vi "Remove UI without races.vi"(8 "error in":errorcluster, 10 "standard events":T1, 11 "sub panel ref in":refnum<vi>) -> (0 "error out":errorcluster, 3 "sub panel ref out":refnum<vi>)   [LabVIEW 2013, in "configuration library.lvlib"]
uses:
  configuration library.lvlib
  <vilib>/NI/Configuration Framework/Node/StandardEvents.ctl
  <vilib>/NI/Configuration Framework/Node/UserEventRef.ctl
  <vilib>/NI/Configuration Framework/Controls/EventCluster.ctl
  <vilib>/NI/Configuration Framework/Node/NodeChangeEvent.ctl
  <vilib>/NI/Configuration Framework/Node/NodeRef.ctl
  <vilib>/NI/Configuration Framework/Node/NISE_CEF_Node.lvclass
  <vilib>/NI/Configuration Framework/Node/CacheState.ctl
  <vilib>/NI/Configuration Framework/Node/RefreshUIEvent.ctl
  <vilib>/NI/Configuration Framework/Node/StopEvent.ctl
  <vilib>/NI/Configuration Framework/NISE_CEF_TreeControl.lvlib
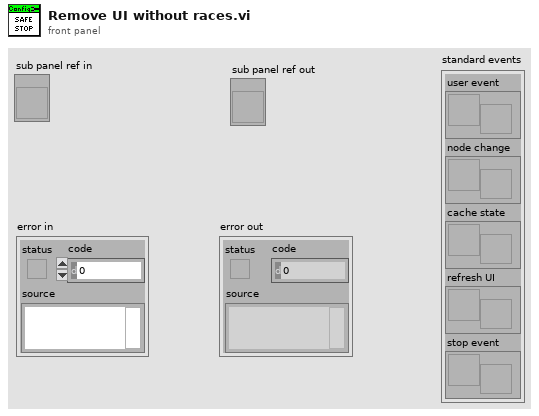
[diagram p1: front panel]
types:
  T1 = typedef "NISE_CEF_Node.lvclass/StandardEvents.ctl" = cluster{"user event":T2, "node change":T3, "cache state":T4, "refresh UI":T5, "stop event":T6}
  T2 = typedef "NISE_CEF_Node.lvclass/UserEventRef.ctl" = refnum<user-event>
  T3 = typedef "NISE_CEF_Node.lvclass/NodeChangeEvent.ctl" = refnum<user-event>
  T4 = typedef "NISE_CEF_Node.lvclass/CacheState.ctl" = refnum<user-event>
  T5 = typedef "NISE_CEF_Node.lvclass/RefreshUIEvent.ctl" = refnum<user-event>
  T6 = typedef "NISE_CEF_Node.lvclass/StopEvent.ctl" = refnum<user-event>
  T7 = typedef "NISE_CEF_TreeControl.lvlib/EventCluster.ctl" = cluster{"command":string, "data":string}
  T8 = enum32{"Bad", "Idle", "Run top level", "Running"}
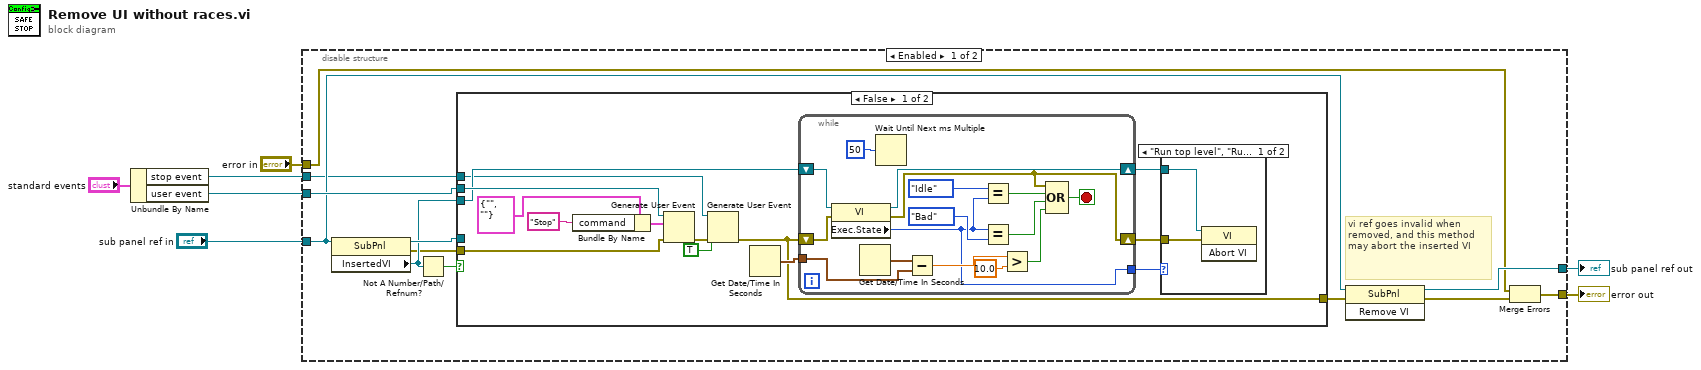
[diagram p0: block diagram]
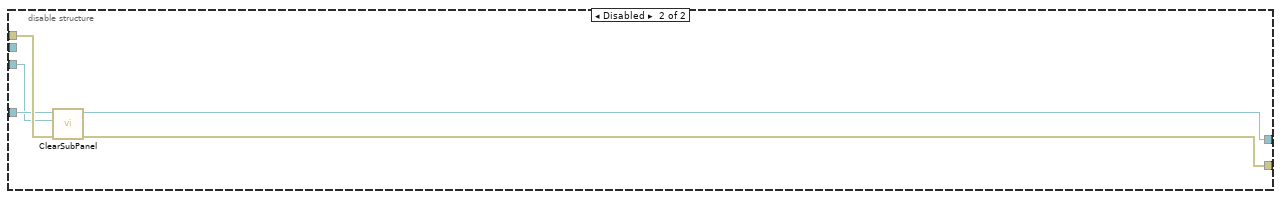
[diagram p4: hidden frame]
diagram:
  n1 = Unbundle By Name("standard events") -> ("stop event"=w1:T6, "user event"=w2:T2)
  n2 = disable-structure shown="Enabled" {
    disable-tunnel: "error in" -> [w12 w57]
    disable-tunnel: "sub panel ref in" -> [w14 w56]
    disable-tunnel: w2 -> [w18 w53]
    disable-tunnel: [w17 w55] -> w5
    disable-tunnel: [w13 w54] -> w4
    disable-tunnel: w1 -> [w8 _]
    frame Enabled {
      # "vi ref goes invalid when removed, and this method may abort the inserted VI"
      n3 = property class="SubPnl"(reference=w14) -> (reference out=w11:refnum<vi>, error out=w9:errorcluster, "InsertedVI"=w10:refnum<vi>)  [unwired: 1 in]
      n4 = Not A Number/Path/Refnum?(number/path/refnum=w10) -> (NaN/Path/Refnum?=w19:bool)
      n5 = case shown="False" w19 {
        tunnel: [w22 w52] -> w16
        tunnel: w10 -> [w28 _]
        tunnel: w9 -> [w23 w52]
        tunnel: w18 -> [w33 _]
        tunnel: w11 -> [_ _]
        tunnel: w8 -> [w21 _]
        frame False {
          n6 = Bundle By Name(cluster=T7 {"command"="", "data"=""} ("event data"), "command"="Stop") -> (w31:T7)
          n7 = Generate User Event(user event=w33, event data cluster=w31, error in=w23) -> (error out=w25:errorcluster)  [unwired: 1 in, 1 out]
          n8 = Generate User Event(user event=w21, event data cluster=TRUE ("event data"), error in=w25) -> (error out=w22:errorcluster)  [unwired: 1 in, 1 out]
          n9 = Get Date/Time In Seconds() -> (seconds since 1Jan1904=w29:timestamp)
          n10 = while {
            tunnel: w29 -> [w48]
            shift-right: [w41] -> w27
            shift-left: w22 -> [w51]
            shift-right: [w37] -> w26
            shift-left: w28 -> [w50]
            tunnel: [w36] -> w24
            stop <- w44 stop-if-true
            n11 = property class="VI"(reference=w50, error in=w51) -> (reference out=w37:refnum<vi>, error out=w41:errorcluster, "Exec.State"=w36:T8)
            n12 = Get Date/Time In Seconds() -> (seconds since 1Jan1904=w49:timestamp)
            n13 = Wait Until Next ms Multiple(millisecond multiple=u32 50 ("milliseconds to wait")) -> ()  [unwired: 1 out]
            n14 = Subtract(x=w49, y=w48) -> (x-y=w47:dbl)
            n15 = Equal?(x=T8."Idle", y=w36) -> (x = y?=w39:bool)
            n16 = Equal?(x=w36, y=T8."Bad") -> (x = y?=w38:bool)
            n17 = Greater?(x=w47, y=10.0) -> (0:w45:bool)
            n18 = Compound Arithmetic op=OR(w41, w39, w38, w45) -> (w44:bool)
          }
          n19 = case shown="\"Run top level\", \"Running\"" w24 {
            tunnel: w27 -> [w35 _]
            tunnel: w26 -> [w34 _]
            frame "Run top level", "Running" {
              n20 = invoke class="VI" method="Abort VI"(reference=w34, error in=w35) -> ()  [unwired: 1 in, 3 out]
            }
            frame "Idle", Default {
            }
          }
        }
        frame True {
          # "Reference is not valid if there is no VI"
        }
      }
      n21 = invoke class="SubPnl" method="Remove VI"(reference=w14, error in=w16) -> (reference out=w17:refnum<vi>, error out=w15:errorcluster)  [unwired: 1 in, 1 out]
      n22 = Merge Errors(w12, w15) -> (w13:errorcluster)
    }
    frame Disabled {
      n23 = call <vilib>:"ClearSubPanel.vi"("error in"=w57, "user event ref"=w53, "sub panel ref in"=w56) -> ("error out"=w54:errorcluster, "sub panel ref out"=w55:refnum<vi>)  [unwired: 7 in]
    }
  }
  "error out" <- w4
  "sub panel ref out" <- w5
